vi "DataToArray.vi"(10 "RFFE_Data":T2 {"Toggle (high to low)" items=["0", "1", "Z", "L", "H", "X", "T", "V"]; "X Array" items=["0", "1", "Z", "L", "H", "X", "T", "V"]; "Z Array" items=["0", "1", "Z", "L", "H", "X", "T", "V"]; "L Array" items=["0", "1", "Z", "L", "H", "X", "T", "V"]; "H Array" items=["0", "1", "Z", "L", "H", "X", "T", "V"]; "One Array" items=["0", "1", "Z", "L", "H", "X", "T", "V"]; "Zero Array" items=["0", "1", "Z", "L", "H", "X", "T", "V"]}, 11 "Value":T1) -> (3 "Data":u8[](array[numeric]))   [LabVIEW 2013]
doc: "This VI converts a signle MIPI sample into a properly sampled array."
uses:
  Ctrls/RFFE_Data.ctl
  Ctrls/ClockDataChannels.ctl
  Ctrls/BitStates.ctl
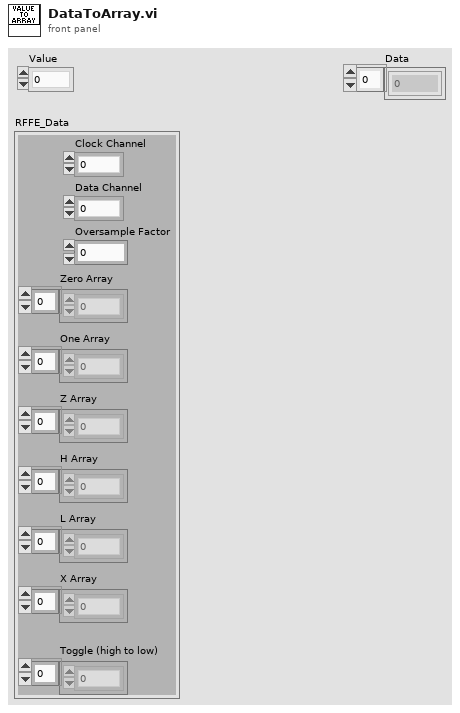
[diagram p1: front panel]
types:
  T1 = typedef "BitStates.ctl" = enum16{"0", "1", "Z", "L", "H", "X", "Toggle"}
  T2 = typedef "RFFE_Data.ctl" = cluster{"Clock Channel":T3, "Data Channel":T3, "Oversample Factor":u8, "Zero Array":u8[], "One Array":u8[], "Z Array ":u8[], "H Array":u8[], "L Array":u8[], "X Array":u8[], "Toggle (high to low)":u8[]}
  T3 = typedef "ClockDataChannels.ctl" = enum16{"0", "1"}
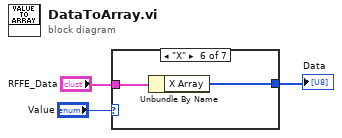
[diagram p0: block diagram]
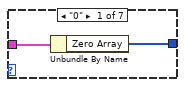
[diagram p2: hidden frame]
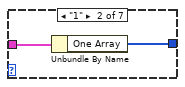
[diagram p3: hidden frame]
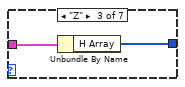
[diagram p4: hidden frame]
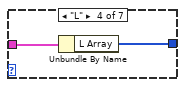
[diagram p5: hidden frame]
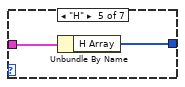
[diagram p6: hidden frame]
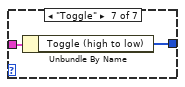
[diagram p7: hidden frame]
diagram:
  n1 = case shown="\"X\"" "Value" {
    tunnel: "RFFE_Data" -> [w5 w7 w9 w11 w13 w15 w17]
    tunnel: [w4 w6 w8 w10 w12 w14 w16] -> w3
    frame "0" {
      n2 = Unbundle By Name(w5) -> ("Zero Array"=w4:u8[])
    }
    frame "1" {
      n3 = Unbundle By Name(w7) -> ("One Array"=w6:u8[])
    }
    frame "Z" {
      n4 = Unbundle By Name(w9) -> ("H Array"=w8:u8[])
    }
    frame "L" {
      n5 = Unbundle By Name(w11) -> ("L Array"=w10:u8[])
    }
    frame "H" {
      n6 = Unbundle By Name(w13) -> ("H Array"=w12:u8[])
    }
    frame "X" {
      n7 = Unbundle By Name(w15) -> ("X Array"=w14:u8[])
    }
    frame "Toggle" {
      n8 = Unbundle By Name(w17) -> ("Toggle (high to low)"=w16:u8[])
    }
  }
  "Data" <- w3
